vi "Task05MainVI.vi"() -> ()   [LabVIEW 2017]
panel:
  out "Numeric":u32
  in  "stop":bool
  in  "Switch Array":bool[](array[boolean])
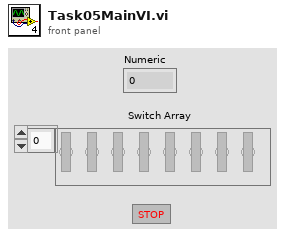
[diagram p1: front panel]
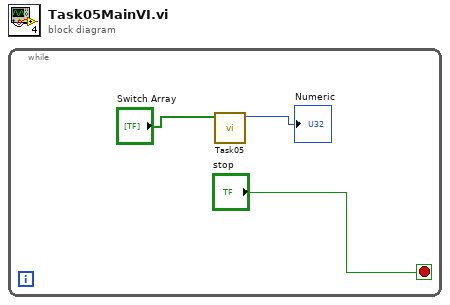
[diagram p0: block diagram]
diagram:
  n1 = while {
    stop <- "stop" stop-if-true
    n2 = call "Task05.vi"("Array"="Switch Array") -> ("Numeric"=→"Numeric":u32)  [unwired: 10 in]
  }
